vi "pyobj.vi"() -> ()   [LabVIEW 2024]
panel:
  out "return value":dbl
  in  "stop":bool
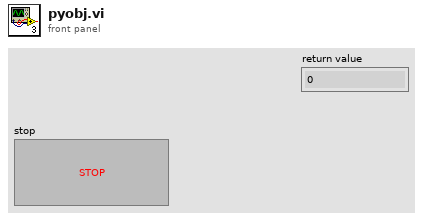
[diagram p1: front panel]
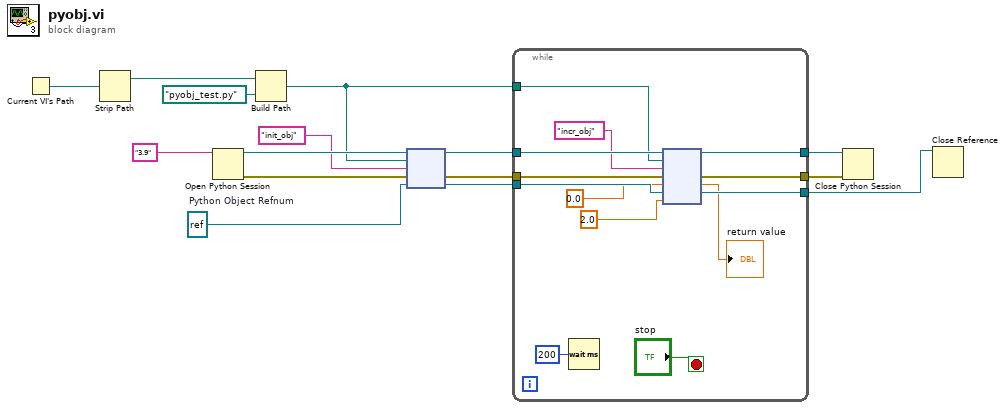
[diagram p0: block diagram]
diagram:
  w8 = refnum<k38> refnum  # Python Object Refnum
  n1 = Current VI's Path() -> (path=w14:path)
  n2 = Strip Path(path=w14) -> (stripped path=w13:path)  [unwired: 1 out]
  n3 = Open Python Session(python version="3.9" ("Python version")) -> (session out=w11:refnum<k35>, error out=w10:errorcluster)  [unwired: 2 in]
  n4 = Build Path(base path=w13, name or relative path=path "pyobj_test.py") -> (appended path=w6:path)
  n5 = node(w11, w6, "init_obj" ("function name"), w10, w8) -> (w7:refnum<k35>, w4:errorcluster, w5:refnum<k38>)  [unwired: 2 out]
  n6 = while {
    tunnel: w7 -> [w28]
    tunnel: [w25] -> w3
    tunnel: w6 -> [w24]
    tunnel: w5 -> [w23]
    tunnel: w4 -> [w22]
    tunnel: [w19] -> w2
    tunnel: [w18] -> w1
    stop <- "stop" stop-if-true
    n7 = Wait (ms)(milliseconds to wait=u32 200) -> ()  [unwired: 1 out]
    n8 = node(w28, w24, "incr_obj" ("function name"), w22, 0.0, w23, 2.0) -> (w25:refnum<k35>, w19:errorcluster, →"return value":dbl, w18:refnum<k38>)  [unwired: 1 in, 2 out]
  }
  n9 = Close Python Session(session in=w3, error in=w2) -> ()  [unwired: 1 out]
  n10 = Close Reference(reference=w1) -> ()  [unwired: 1 in, 1 out]
